vi "Format Text Indicators.vi"(8 "Preferred Exec System":T1(ring), 9 "Priority":T2(ring), 10 "Reentrancy Type":T3(ring), 11 "Reentrant?":bool) -> (0 "Preferred Exec System String":string, 1 "Priority String":string, 2 "Reentrancy String":string)   [LabVIEW 2020, in "VI Properties Editor.lvlib"]
doc: "Formats the reentrancy, priority, and preferred execution system properties into strings to be displayed."
uses:
  VI Properties Editor.lvlib
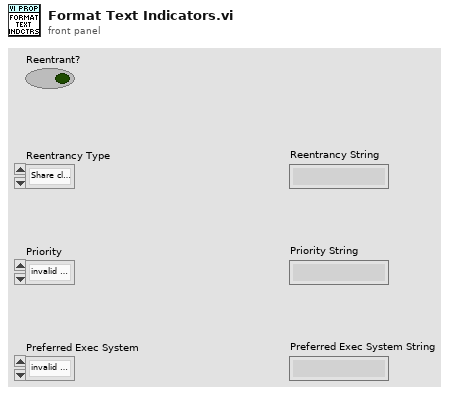
[diagram p1: front panel]
types:
  T1 = enum32{"invalid execution system", "user interface", "standard", "instrument i/o", "data acquisition", "other 1", "other 2", "same as caller"}
  T2 = enum32{"invalid priority", "background priority", "normal priority", "above normal priority", "high priority", "time critical priority", "subroutine"}
  T3 = enum16{"Share clones between instances", "Preallocate clone for each instance"}
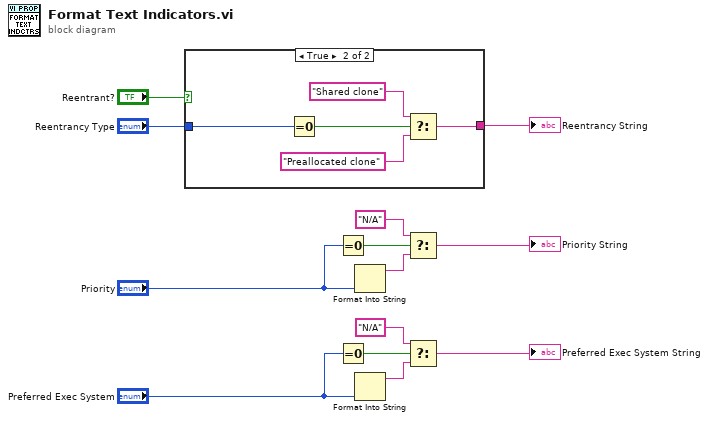
[diagram p0: block diagram]
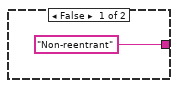
[diagram p2: hidden frame]
diagram:
  n1 = case shown="True" "Reentrant?" {
    tunnel: "Reentrancy Type" -> [_ w19]
    tunnel: ["Non-reentrant" w15] -> w11
    frame False {
    }
    frame True {
      n2 = Equal To 0?(x=w19) -> (x = 0?=w18:bool)
      n3 = Select(t="Shared clone", s=w18, f="Preallocated clone") -> (s? t:f=w15:string)
    }
  }
  "Reentrancy String" <- w11
  n4 = Equal To 0?(x="Priority") -> (x = 0?=w9:bool)
  n5 = Equal To 0?(x="Preferred Exec System") -> (x = 0?=w4:bool)
  n6 = Format Into String("Priority") -> (resulting string=w7:string)  [unwired: 3 in, 1 out]
  n7 = Format Into String("Preferred Exec System") -> (resulting string=w5:string)  [unwired: 3 in, 1 out]
  n8 = Select(t="N/A", s=w9, f=w7) -> (s? t:f=→"Priority String":string)
  n9 = Select(t="N/A", s=w4, f=w5) -> (s? t:f=→"Preferred Exec System String":string)
